vi "Ejercicio_Pots.vi"() -> ()   [LabVIEW 2016]
uses:
  <vilib>/DAQmx/read.llb/DAQmx Read (Analog 1D DBL NChan 1Samp).vi
  <vilib>/DAQmx/create/channels.llb/DAQmx Create Channel (AI-Voltage-Basic).vi
  <vilib>/DAQmx/configure/timing.llb/DAQmx Timing (Sample Clock).vi
  <vilib>/DAQmx/miscellaneous.llb/DAQmx Fill In Error Info.vi
panel:
  out "POT 3":dbl(knob) scale=0.0..359.0
  out "POT 2":dbl(knob) scale=0.0..359.0
  out "POT 1":dbl(knob) scale=0.0..359.0
  out "XY Graph":cluster{dbl[], dbl[]}(graph)
  in  "L3":dbl(slide) scale=0.0..3.0
  in  "L2":dbl(slide) scale=0.0..3.0
  in  "L1":dbl(slide) scale=0.0..3.0
  in  "Stop Button":bool
  out "cluster":T1
  out "data":dbl[](graph)
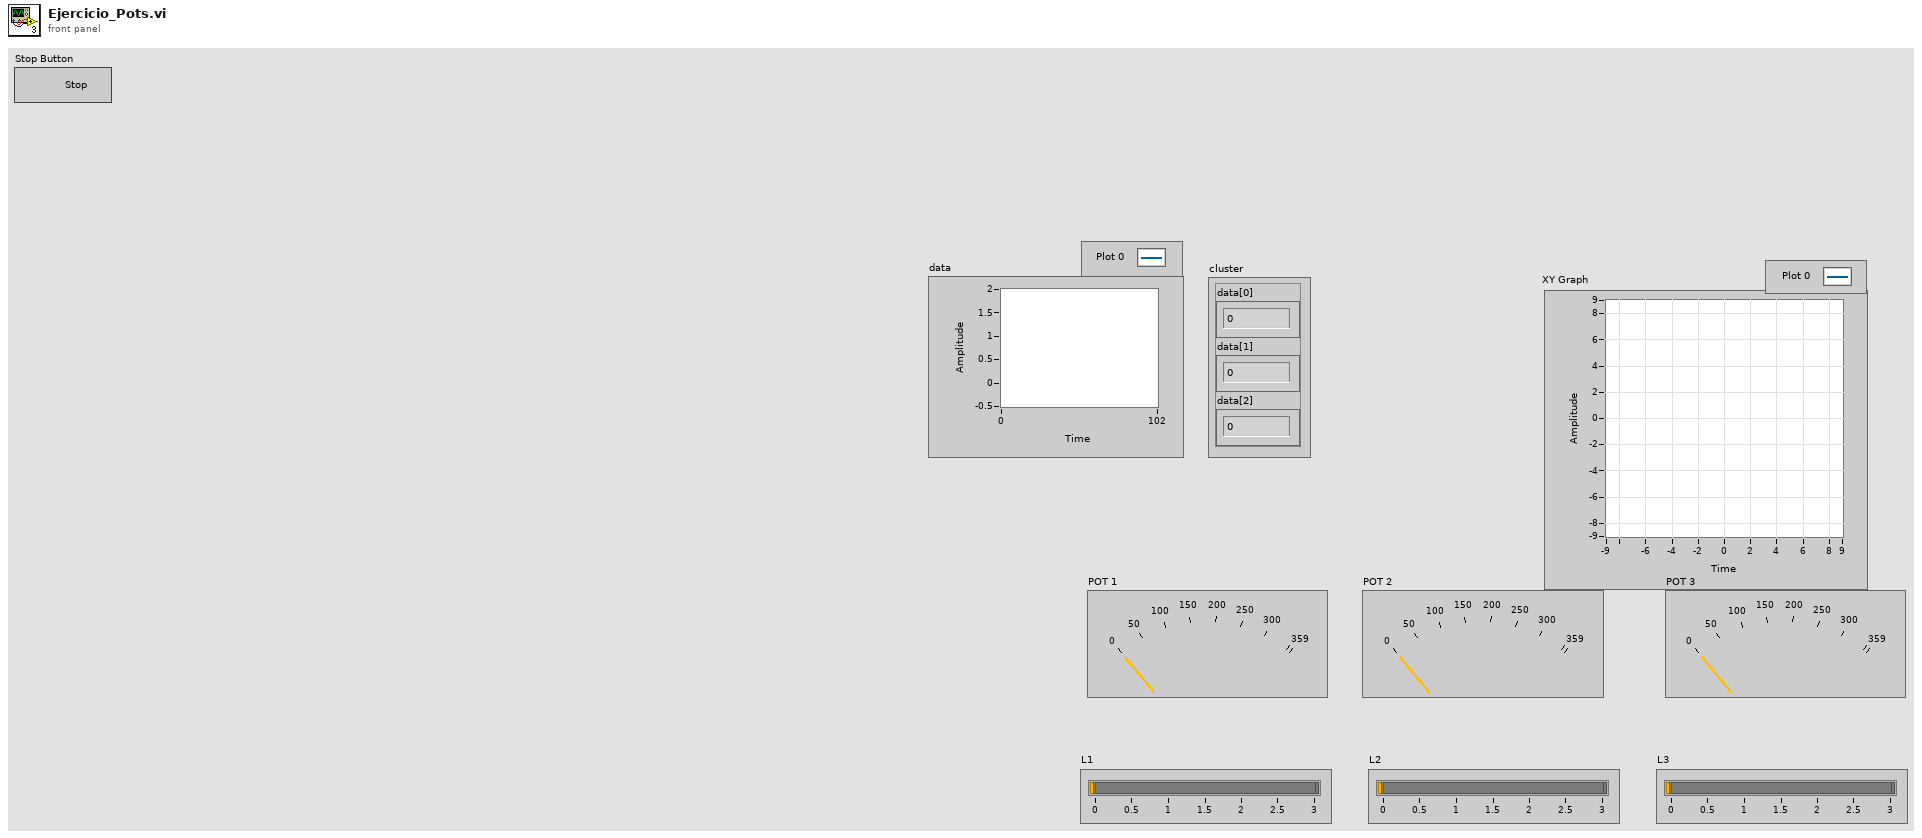
[diagram p1: front panel]
types:
  T1 = cluster{"data[0]":dbl, "data[1]":dbl, "data[2]":dbl, "data[3]":dbl, "data[4]":dbl, "data[5]":dbl, "data[6]":dbl, "data[7]":dbl, "data[8]":dbl}
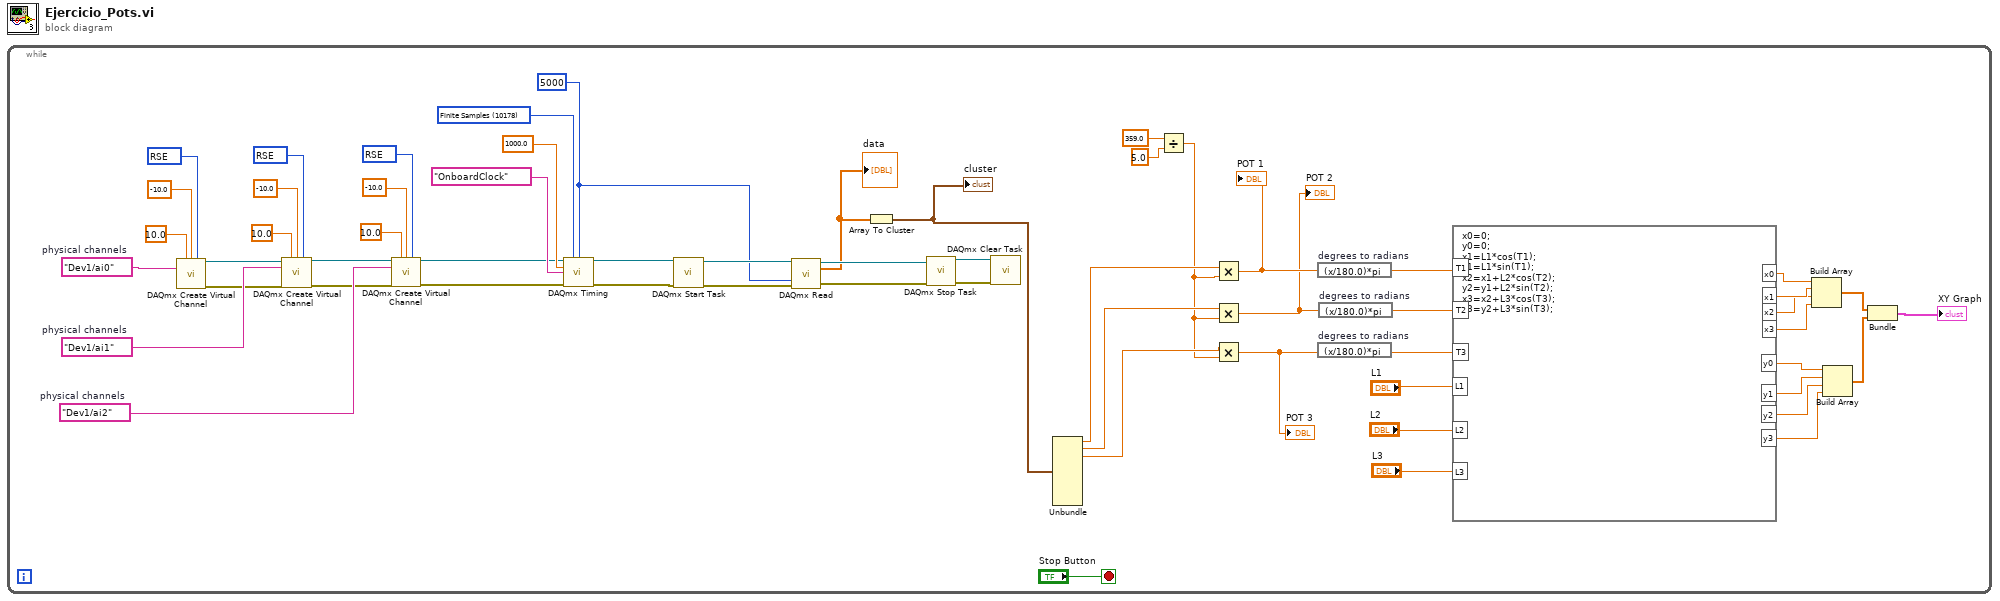
[diagram p0: block diagram]
diagram:
  n1 = while {
    stop <- "Stop Button" stop-if-true
    w36 = tag "Dev1/ai2"  # physical channels
    w39 = 10083 items=["Default"=-1, "RSE"=10083, "NRSE"=10078, "Differential"=10106, "Pseudodifferential"=12529] ("input terminal configuration")
    w40 = tag "Dev1/ai1"  # physical channels
    w43 = 10083 items=["Default"=-1, "RSE"=10083, "NRSE"=10078, "Differential"=10106, "Pseudodifferential"=12529] ("input terminal configuration")
    w48 = 5000 ("samples per channel")
    w55 = 10178 items=["Finite Samples"=10178, "Continuous Samples"=10123, "Hardware Timed Single Point"=12522] ("sample mode")
    w56 = tag "Dev1/ai0"  # physical channels
    w59 = 10083 items=["Default"=-1, "RSE"=10083, "NRSE"=10078, "Differential"=10106, "Pseudodifferential"=12529] ("input terminal configuration")
    n2 = call-poly <vilib>:"DAQmx Create Virtual Channel.vi"("maximum value"=10.0, "minimum value"=-10.0, "input terminal configuration"=w59, "physical channels"=w56) -> ("task out"=w34:refnum<k21>, "error out"=w33:errorcluster)  [unwired: 10 in]
    n3 = call-poly <vilib>:"DAQmx Create Virtual Channel.vi"("task in"=w34, "maximum value"=10.0, "minimum value"=-10.0, "input terminal configuration"=w43, "physical channels"=w40, "error in"=w33) -> ("task out"=w35:refnum<k21>, "error out"=w32:errorcluster)  [unwired: 8 in]
    n4 = call-poly <vilib>:"DAQmx Create Virtual Channel.vi"("task in"=w35, "maximum value"=10.0, "minimum value"=-10.0, "input terminal configuration"=w39, "physical channels"=w36, "error in"=w32) -> ("task out"=w30:refnum<k21>, "error out"=w31:errorcluster)  [unwired: 8 in]
    n5 = call-poly <vilib>:"DAQmx Timing.vi"("task/channels in"=w30, "sample mode"=w55, "samples per channel"=w48, "rate"=1000.0, "source"=tag "OnboardClock", "error in"=w31) -> ("task out"=w52:refnum<k21>, "error out"=w50:errorcluster)  [unwired: 8 in]
    n6 = call <vilib>:"DAQmx Start Task.vi"("task/channels in"=w52, "error in"=w50) -> ("task out"=w51:refnum<k21>, "error out"=w49:errorcluster)  [unwired: 12 in]
    n7 = call-poly <vilib>:"DAQmx Read.vi"("task/channels in"=w51, "timeout"=w48, "error in"=w49) -> ("task out"=w46:refnum<k21>, "data"=w29:dbl[], "error out"=w47:errorcluster)  [unwired: 10 in]
    "data" <- w29
    n8 = Array To Cluster(array=w29) -> (cluster=w27:T1)
    "cluster" <- w27
    n9 = call <vilib>:"DAQmx Stop Task.vi"("task/channels in"=w46, "error in"=w47) -> ("task out"=w45:refnum<k21>, "error out"=w44:errorcluster)  [unwired: 12 in]
    n10 = call <vilib>:"DAQmx Clear Task.vi"("task in"=w45, "error in"=w44) -> ()  [unwired: 13 in, 1 out]
    n11 = Unbundle(w27) -> ("data[0]"=w7:dbl, "data[1]"=w8:dbl, "data[2]"=w9:dbl)  [unwired: 6 out]
    n12 = Divide(x=359.0, y=5.0) -> (x/y=w4:dbl)
    n13 = Multiply(x=w7, y=w4) -> (x*y=w3:dbl)
    "POT 1" <- w3
    n14 = Multiply(x=w8, y=w4) -> (x*y=w2:dbl)
    "POT 2" <- w2
    n15 = Multiply(x=w9, y=w4) -> (x*y=w1:dbl)
    "POT 3" <- w1
    n16 = expression code="(x/180.0)*pi" "degrees to radians"(w3) -> (w26:dbl)
    n17 = expression code="(x/180.0)*pi" "degrees to radians"(w1) -> (w15:dbl)
    n18 = expression code="(x/180.0)*pi" "degrees to radians"(w2) -> (w14:dbl)
    n19 = formula code="x0=0;\ny0=0;\nx1=L1*cos(T1);\ny1=L1*sin(T1);\nx2=x1+L2*cos(T2);\ny2=y1+L2*sin(T2);\nx3=x2+L3*cos(T3);\ny3=y2+L3*sin(T3);"("T1"=w26, "L1"="L1", "T2"=w14, "T3"=w15, "L2"="L2", "L3"="L3") -> ("x0"=w24:dbl, "x1"=w23:dbl, "y0"=w22:dbl, "y1"=w21:dbl, "x2"=w11:dbl, "x3"=w10:dbl, "y2"=w13:dbl, "y3"=w12:dbl)
    n20 = Build Array(w24, w23, w11, w10) -> (w20:dbl[])
    n21 = Build Array(w22, w21, w13, w12) -> (w19:dbl[])
    n22 = Bundle(w20, w19) -> (→"XY Graph":cluster{dbl[], dbl[]})  [unwired: 1 in]
  }
